vi "Deserialise content.vi"(8 "error in (no error)":errorcluster, 10 "JSON String to decode":string, 11 "object in":refnum<class "Message Class.lvclass">) -> (0 "error out":errorcluster, 3 "object out":refnum<class "Message Class.lvclass">)   [LabVIEW 2018, in "ClientMessaging.lvlib" / "Message Class.lvclass"]
doc: "Deserialise a string with metadata"
uses:
  Message Class.lvclass
  Message Class.lvclass/Message Class.ctl
  <vilib>/addons/_JKI.lib/Serialization/JSON/JKI JSON Serialization.lvlib
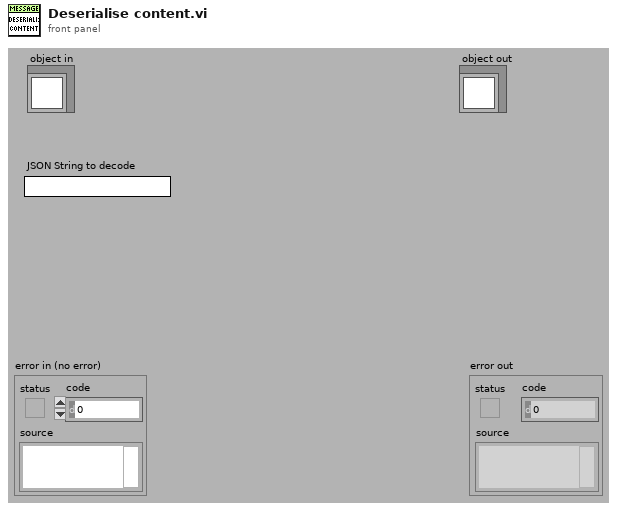
[diagram p1: front panel]
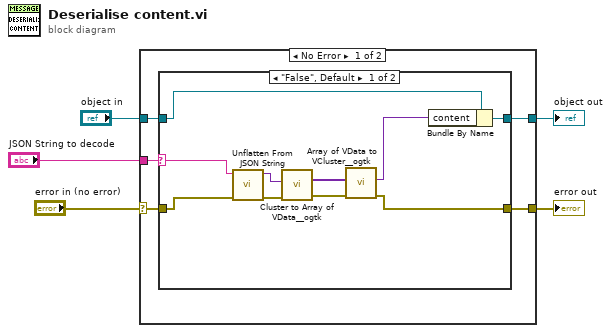
[diagram p0: block diagram]
diagram:
  n1 = case shown="No Error" "error in (no error)" {
    selector: "error in (no error)" -> [w8 w24]
    tunnel: [w7 w24] -> w4
    tunnel: [w9 w23] -> w2
    tunnel: "object in" -> [w10 w23]
    tunnel: "JSON String to decode" -> [w6 _]
    frame No Error {
      n2 = case shown="\"False\", Default" w6 {
        selector: w6 -> [w18 _]
        tunnel: w10 -> [w20 w22]
        tunnel: [w19 w22] -> w9
        tunnel: w8 -> [w17 w21]
        tunnel: [w12 w21] -> w7
        frame "False", Default {
          n3 = call <vilib>:"Unflatten From JSON String.vi"("error in (no error)"=w17, "JSON String"=w18) -> ("error out"=w16:errorcluster, "Variant"=w15:variant)  [unwired: 8 in]
          n4 = call <userlib>:"Cluster to Array of VData__ogtk.vi"("error in (no error)"=w16, "Cluster"=w15) -> ("error out"=w14:errorcluster, "Array of VData"=w11:variant[])  [unwired: 8 in]
          n5 = call <userlib>:"Array of VData to VCluster__ogtk.vi"("error in (no error)"=w14, "Array"=w11) -> ("error out"=w12:errorcluster, "VCluster"=w13:variant)  [unwired: 8 in]
          n6 = Bundle By Name(cluster=w20, "content"=w13) -> (w19:refnum<class "Message Class.lvclass">)
        }
        frame "" {
        }
      }
    }
    frame Error {
    }
  }
  "error out" <- w4
  "object out" <- w2
